vi "Thread.Set Processor.vi"(10 "Processor":i32, 11 "Thread in":refnum<class "Thread.lvclass">) -> (3 "Thread out":refnum<class "Thread.lvclass">)   [LabVIEW 2017, in "Thread.lvclass"]
uses:
  Thread.lvclass
  Thread.lvclass/Thread.ctl
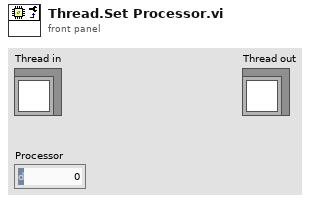
[diagram p1: front panel]
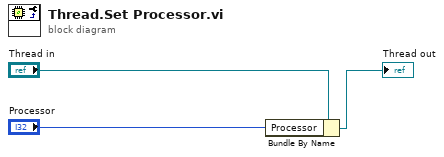
[diagram p0: block diagram]
diagram:
  n1 = Bundle By Name(cluster="Thread in", "Processor"="Processor") -> (→"Thread out":refnum<class "Thread.lvclass">)
